vi "Debug_Log_Control.vi"(0 "Device Selected":u32, 1 "Source":u8 format="%x", 2 "Destination":u8 format="%x", 5 "Enable Log":bool, 7 "Standalone?":bool, 9 "GEA2 Reference In":refnum<k24>, 11 "Error In":errorcluster) -> (10 "GEA2 Reference Out":refnum<k24>, 15 "Error Out":errorcluster)   [LabVIEW 2014]
doc: "This standalone VI sends a GEA2 message to the destination you specify."
uses:
  Common/LabVIEW GEA2 Toolkit/LabVIEW_GEA2_Toolkit.lvlibp
  C:/Automation/DLLs/PC Tools .NET/GeaCommunication.dll
panel:
  # "Enable or disable Debug Log (74)\nand Raw Data Log (41)"
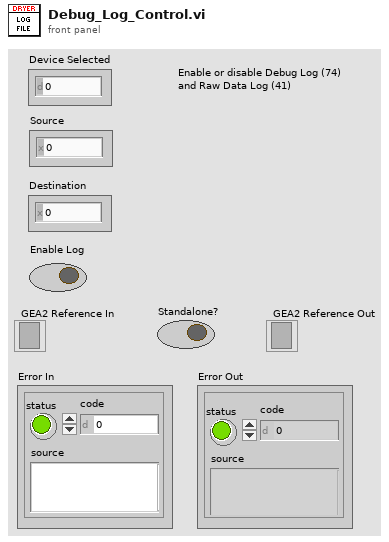
[diagram p1: front panel]
types:
  T1 = cluster{"Source":u8, "Destination":u8, "Command":u8, string}
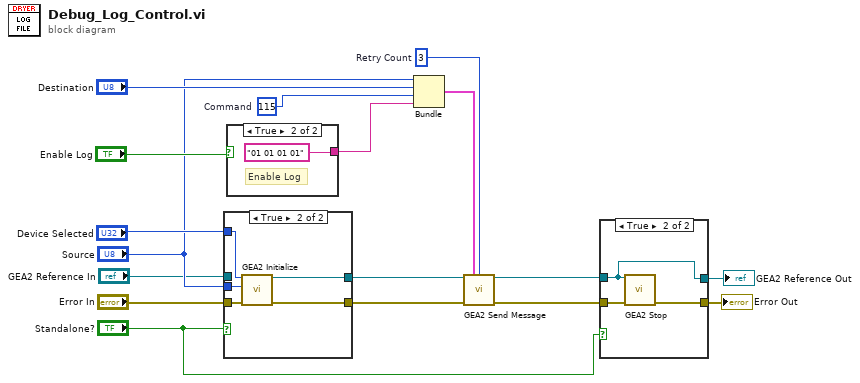
[diagram p0: block diagram]
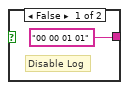
[diagram p4: hidden frame]
diagram:
  w11 = u32 3  # Retry Count
  w8 = u8 115  # Command
  n1 = case shown="True" "Standalone?" {
    tunnel: [w18 w24] -> w17
    tunnel: [w19 w23] -> w14
    tunnel: "Error In" -> [w19 w22]
    tunnel: "Source" -> [_ w21]
    tunnel: "Device Selected" -> [_ w20]
    tunnel: "GEA2 Reference In" -> [w18 _]
    frame False {
    }
    frame True {
      n2 = call "GEA2 Initialize.vi"("Board Index"=w20, "Source Address"=w21, "error in"=w22) -> ("GEA2 Reference Out"=w24:refnum<k24>, "error out"=w23:errorcluster)  [unwired: 10 in, 1 out]
    }
  }
  n3 = case shown="True" "Enable Log" {
    tunnel: ["00 00 01 01" "01 01 01 01"] -> w7
    frame False {
      # "Disable Log"
    }
    frame True {
      # "Enable Log"
    }
  }
  n4 = Bundle("Source"="Source", "Destination"="Destination", "Command"=w8, w7) -> (w10:T1)  [unwired: 1 in]
  n5 = call "GEA2 Send Message.vi"("GEA2 Reference In"=w17, "Input Data"=w10, "# of Tries"=w11, "Error In"=w14) -> ("GEA2 Reference Out"=w16:refnum<k24>, "Error Out"=w15:errorcluster)  [unwired: 10 in]
  n6 = case shown="True" "Standalone?" {
    tunnel: w16 -> [w28 w29]
    tunnel: w15 -> [w27 w31]
    tunnel: [w27 w30] -> w12
    tunnel: [w28 w29] -> w1
    frame False {
    }
    frame True {
      n7 = call "GEA2 Stop.vi"("GEA2 Reference In"=w29, "Error In"=w31) -> ("Error Out"=w30:errorcluster)  [unwired: 13 in]
    }
  }
  "Error Out" <- w12
  "GEA2 Reference Out" <- w1
